vi "IncrementSequenceNumber.vi"(11 "In":i32) -> (3 "Out":i32)   [LabVIEW 2009]
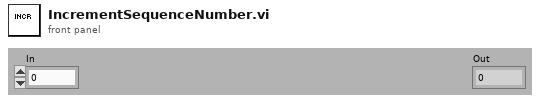
[diagram p1: front panel]
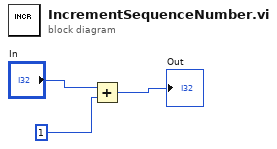
[diagram p0: block diagram]
diagram:
  n1 = Add(x="In", y=1) -> (x+y=→"Out":i32)
